vi "Points_For_arrow_Overlay.vi"(6 "Distances":sgl[](array[numeric]), 7 "AvgMinMax":enum16{"Average", "Max", "Min", "Max2"}(ring), 8 "error in (no error)":errorcluster, 9 "Search Lines":T1[](array[typedef]) {"Edge Info"."Distance (Real-World)" format="%.2f"; "Edge Info"."Location (Real-World)"."Y" format="%.2g"; "Edge Info"."Location (Real-World)"."X" format="%.2f"; "Edge Info"."Noise" format="%.2f"; "Edge Info"."Location (Pixel)"."Y" format="%.2g"; "Edge Info"."Location (Pixel)"."X" format="%.2f"; "Edge Info"."Strength" format="%.2f"; "Edge Info"."Distance (Pixel)" format="%.2f"}, 10 "Last Edges":T2[](array[typedef]) {"Distance (Real-World)" format="%.2f"; "Location (Real-World)"."Y" format="%.2g"; "Location (Real-World)"."X" format="%.2f"; "Noise" format="%.2f"; "Location (Pixel)"."Y" format="%.2g"; "Location (Pixel)"."X" format="%.2f"; "Strength" format="%.2f"; "Distance (Pixel)" format="%.2f"}, 11 "First Edges":T2[](array[typedef]) {"Distance (Real-World)" format="%.2f"; "Location (Real-World)"."Y" format="%.2g"; "Location (Real-World)"."X" format="%.2f"; "Noise" format="%.2f"; "Location (Pixel)"."Y" format="%.2g"; "Location (Pixel)"."X" format="%.2f"; "Strength" format="%.2f"; "Distance (Pixel)" format="%.2f"}) -> (0 "error out":errorcluster, 3 "Points For Array Overlay":cluster{"X":sgl, "Y":sgl}[](array[cluster]))   [LabVIEW 2019, in "Algorithm.lvclass"]
uses:
  FrameworkOverrides/Algorithm.lvclass
  <vilib>/vision/Measure.llb/Edge New.ctl
  <vilib>/vision/Measure.llb/Search Line.ctl
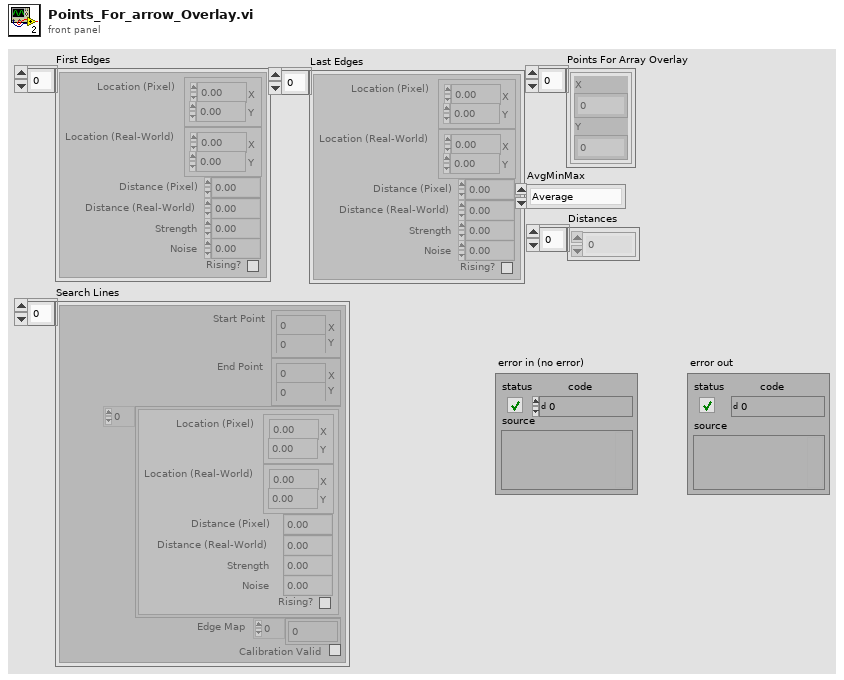
[diagram p1: front panel]
types:
  T1 = typedef "Search Line.ctl" = cluster{"Start Point":cluster{"X":sgl, "Y":sgl}, "End Point":cluster{"X":sgl, "Y":sgl}, "Edge Info":T2[], "Edge Map":dbl[], "Calibration Valid":bool}
  T2 = typedef "Edge New.ctl" = cluster{"Location (Pixel)":cluster{"X":sgl, "Y":sgl}, "Location (Real-World)":cluster{"X":sgl, "Y":sgl}, "Distance (Pixel)":dbl, "Distance (Real-World)":dbl, "Strength":dbl, "Noise":dbl, "Rising?":bool}
  T3 = cluster{"Start Point":cluster{"X":sgl, "Y":sgl}, "Location (Pixel)":cluster{"X":sgl, "Y":sgl}, "Location (Pixel)":cluster{"X":sgl, "Y":sgl}, "End Point":cluster{"X":sgl, "Y":sgl}}
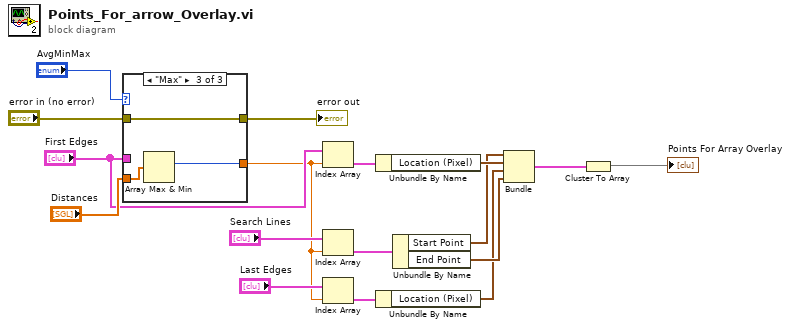
[diagram p0: block diagram]
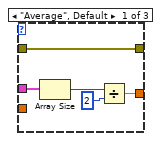
[diagram p2: hidden frame]
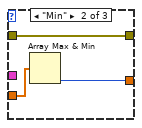
[diagram p3: hidden frame]
diagram:
  n1 = case shown="\"Max\"" "AvgMinMax" {
    tunnel: "Distances" -> [_ w25 w28]
    tunnel: [w19 w24 w27] -> w5
    tunnel: "First Edges" -> [w22 _ _]
    tunnel: "error in (no error)" -> [w18 w23 w26]
    tunnel: [w18 w23 w26] -> w3
    frame "Average", Default {
      n2 = Array Size(array=w22) -> (size(s)=w21:i32)
      n3 = Divide(x=w21, y=2) -> (x/y=w19:dbl)
    }
    frame "Min" {
      n4 = Array Max & Min(array=w25) -> (min index (indices)=w24:i32)  [unwired: 3 out]
    }
    frame "Max" {
      n5 = Array Max & Min(array=w28) -> (max index (indices)=w27:i32)  [unwired: 3 out]
    }
  }
  "error out" <- w3
  n6 = Index Array(array="First Edges", index=w5) -> (element=w13:T2)
  n7 = Index Array(array="Search Lines", index=w5) -> (element=w15:T1)
  n8 = Index Array(array="Last Edges", index=w5) -> (element=w14:T2)
  n9 = Unbundle By Name(w13) -> ("Location (Pixel)"=w11:cluster{"X":sgl, "Y":sgl})
  n10 = Unbundle By Name(w14) -> ("Location (Pixel)"=w10:cluster{"X":sgl, "Y":sgl})
  n11 = Unbundle By Name(w15) -> ("Start Point"=w2:cluster{"X":sgl, "Y":sgl}, "End Point"=w12:cluster{"X":sgl, "Y":sgl})
  n12 = Bundle("Start Point"=w2, "Location (Pixel)"=w11, "Location (Pixel)"=w10, "End Point"=w12) -> (w9:T3)  [unwired: 1 in]
  n13 = Cluster To Array(cluster=w9) -> (array=→"Points For Array Overlay":cluster{"X":sgl, "Y":sgl}[])
